vi "InitWebsocketMessageBroker.vi"(8 "error in (no error)":errorcluster, 9 "Websocket Client Handler":refnum<class "Websocket Client Handler.lvclass">, 10 "Listen Port":u16, 11 "Broker Name":string) -> (0 "error out":errorcluster, 2 "Broadcast Message Transport":refnum<class "Message Transport Queue.lvclass">, 3 "Websocket Message Broker Interface Ref out":refnum<class "Websocket Message Broker Interface Ref.lvclass">)   [LabVIEW 2016, in "Stream Mediator.lvlib" / "Websocket Message Broker Interface Ref.lvclass"]
doc: "--\nCopyright © 2017 Composed SystemsI All rights reserved.\n\nAuthor: Jon McBee <jon.mcbee@composed.io>\n\nThis library is provided \"AS IS\" ,WITHOUT WARRANTIES OR\nCONDITIONS OF ANY KIND, either express or implied.\n\nComposed Systems -- composed.io\n\nStream 0.0.1.1\nJon McBee - Composed Systems\nCopyright (c) 2017, Composed Systems"
uses:
  <userlib>/Composed Systems/Stream/Mediator/Classes/Websocket Message Broker Interface Ref/Websocket Message Broker Interface Ref.lvclass
  C:/Program Files (x86)/National Instruments/LabVIEW 2016/user.lib/Composed Systems/Stream/Mediator/Classes/Message Broker Interface Ref/Message Broker Interface Ref.lvclass
  C:/Program Files (x86)/National Instruments/LabVIEW 2016/user.lib/Composed Systems/Stream/Mediator/Classes/Message Broker Interface/Message Broker Interface.lvclass
  <userlib>/Composed Systems/Stream/Mediator/Classes/Websocket Client Handler Actor/Websocket Client Handler/Websocket Client Handler.lvclass
  <userlib>/Composed Systems/Stream/Mediator/Classes/Message Transport Queue/Message Transport Queue.lvclass
  <userlib>/Composed Systems/Stream/Mediator/Classes/Websocket Topic Actor/Websocket Topic Actor.lvclass
  <userlib>/Composed Systems/Stream/Mediator/Classes/Websocket Server Actor/Websocket Server/Websocket Server.lvclass
  C:/Program Files (x86)/National Instruments/LabVIEW 2016/user.lib/Composed Systems/Stream/Mediator/Classes/Mediated Asynchronous Actor/Mediated Asynchronous Actor.lvclass
  <userlib>/Composed Systems/Stream/Mediator/Classes/Websocket Server Actor/Websocket Server/Websocket Server.lvclass/Websocket Server.ctl
  <userlib>/Composed Systems/Stream/Mediator/Classes/Websocket Message Broker Interface Ref/Websocket Message Broker Interface Ref.lvclass/Websocket Message Broker Interface Ref.ctl
  <userlib>/Composed Systems/Stream/Mediator/Classes/Websocket Message Broker/Websocket Message Broker.lvclass
  C:/Program Files (x86)/National Instruments/LabVIEW 2016/user.lib/Composed Systems/Stream/Mediator/Classes/Message Broker/Message Broker.lvclass
  <userlib>/Composed Systems/Stream/Mediator/Classes/Message Broker Interface Ref/Message Broker Interface Ref.lvclass
  <userlib>/Composed Systems/Stream/Mediator/Classes/Mediated Asynchronous Actor/Mediated Asynchronous Actor.lvclass
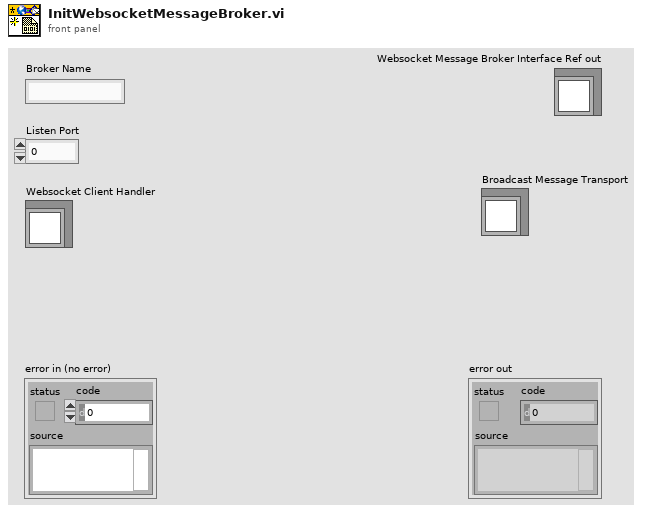
[diagram p1: front panel]
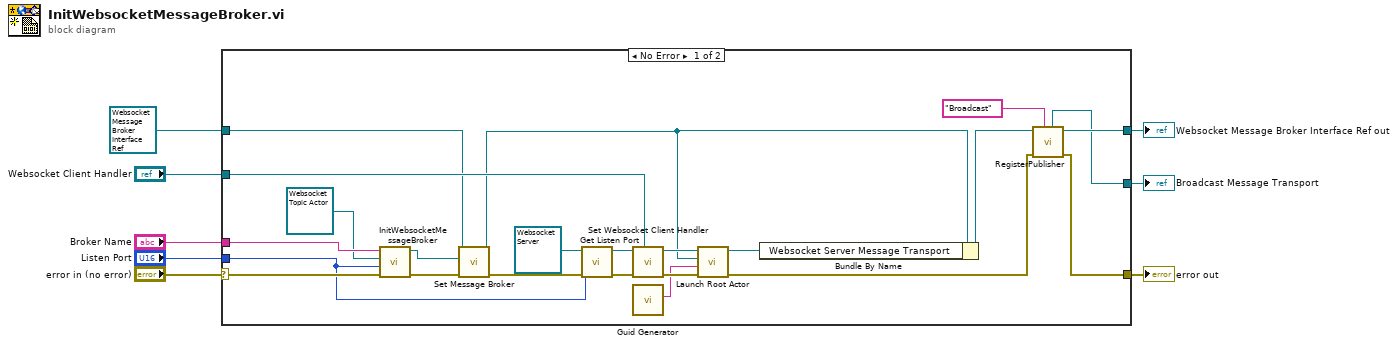
[diagram p0: block diagram]
diagram:
  n1 = case shown="No Error" "error in (no error)" {
    selector: "error in (no error)" -> [w31 w33]
    tunnel: [w10 w33] -> w7
    tunnel: [w13 w32] -> w5
    tunnel: refnum<class "Websocket Message Broker Interface Ref.lvclass"> refnum ("Websocket Message Broker Interface Ref in") -> [w20 w32]
    tunnel: "Broker Name" -> [w30 _]
    tunnel: "Listen Port" -> [w15 _]
    tunnel: "Websocket Client Handler" -> [w26 _]
    tunnel: [w9 _] -> w1
    frame No Error {
      n2 = call <userlib>:"InitWebsocketMessageBroker.vi"("error in (no error)"=w31, "Listen Port"=w15, "Websocket Topic Actor"=refnum<class "Websocket Topic Actor.lvclass"> refnum, "Broker Name"=w30) -> ("error out"=w28:errorcluster, "Message Broker Ref"=w27:refnum<data-value>)  [unwired: 6 in]
      n3 = call <userlib>:"Set Message Broker.vi"("error in (no error)"=w28, "Broker"=w27, "Message Broker Interface Ref in"=w20) -> ("error out"=w19:errorcluster, "Message Broker Interface Ref out"=w21:refnum<class "Websocket Message Broker Interface Ref.lvclass">)  [unwired: 7 in]
      n4 = call <userlib>:"Get Listen Port.vi"("error in (no error)"=w19, "Listen Port"=w15, "Websocket Server in"=refnum<class "Websocket Server.lvclass"> refnum ("Websocket Server.lvclass")) -> ("error out"=w18:errorcluster, "Websocket Server out"=w16:refnum<class "Websocket Server.lvclass">)  [unwired: 7 in]
      n5 = call <userlib>:"Set Websocket Client Handler.vi"("Websocket Client Handler"=w26, "error in (no error)"=w18, "Websocket Server in"=w16) -> ("error out"=w24:errorcluster, "Websocket Server out"=w22:refnum<class "Websocket Server.lvclass">)  [unwired: 7 in]
      n6 = call <vilib>:"Guid Generator.vi"() -> ("GUID"=w14:string)  [unwired: 10 in, 1 out]
      n7 = call <userlib>:"Launch Root Actor.vi"("error in (no error)"=w24, "Actor Name"=w14, "Message Broker"=w21, "Mediated Asynchronous Actor in"=w22) -> ("error out"=w11:errorcluster, "Command Actor Message Transport"=w23:refnum<class "Message Transport Interface.lvclass">)  [unwired: 6 in]
      n8 = Bundle By Name(cluster=w21, "Websocket Server Message Transport"=w23) -> (w25:refnum<class "Websocket Message Broker Interface Ref.lvclass">)
      n9 = call-dynamic "RegisterPublisher.vi"("Topic Name"="Broadcast", "error in (no error)"=w11, "Message Broker Interface Ref in"=w25) -> ("error out"=w10:errorcluster, "Message Broker Interface Ref out"=w13:refnum<class "Websocket Message Broker Interface Ref.lvclass">, "Transport"=w9:refnum<class "Message Transport Queue.lvclass">)  [unwired: 4 in, 2 out]
    }
    frame Error {
    }
  }
  "error out" <- w7
  "Websocket Message Broker Interface Ref out" <- w5
  "Broadcast Message Transport" <- w1
